vi "Walk Map.vi"(8 "error in (no error)":errorcluster, 11 "Map in":refnum<class "Maze.lvclass">) -> (3 "Map out":refnum<class "Maze.lvclass">)   [LabVIEW 2020, in "Maze.lvclass"]
uses:
  Maze.lvclass
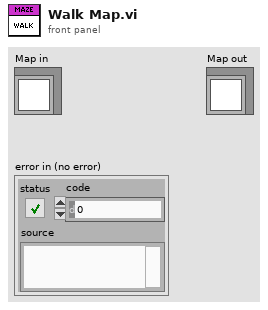
[diagram p1: front panel]
types:
  T1 = typedef "Maze.lvclass/Position.ctl" = cluster{"Row":u64, "Col":u64, "Next Move":enum16{"North", "East", "South", "West", "Halt"}}
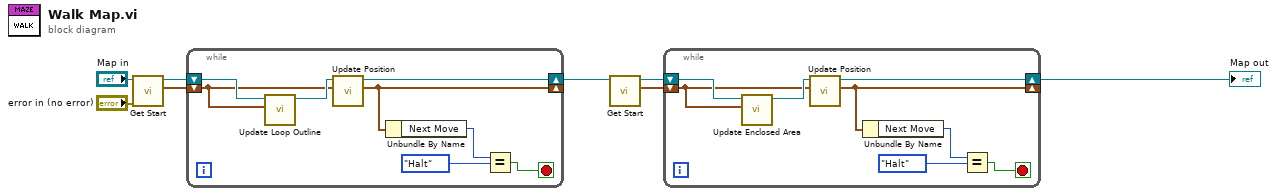
[diagram p0: block diagram]
diagram:
  n1 = call "Get Start.vi"("error in (no error)"="error in (no error)", "Map in"="Map in") -> ("Start Vectors"=w8:T1, "Map out"=w7:refnum<class "Maze.lvclass">)  [unwired: 7 in, 1 out]
  n2 = while {
    shift-right: [w15] -> _
    shift-left: w8 -> [w9]
    shift-right: [w12] -> w1
    shift-left: w7 -> [w11]
    stop <- w13 stop-if-true
    n3 = call "Update Loop Outline.vi"("Start Vectors"=w9, "Map in"=w11) -> ("Map out"=w10:refnum<class "Maze.lvclass">)  [unwired: 9 in]
    n4 = call "Update Position.vi"("Current"=w9, "Map In"=w10) -> ("Next"=w15:T1, "Map Out"=w12:refnum<class "Maze.lvclass">)  [unwired: 6 in, 2 out]
    n5 = Unbundle By Name(w15) -> ("Next Move"=w14:enum16{"North", "East", "South", "West", "Halt"})
    n6 = Equal?(x=w14, y=enum16{"North", "East", "South", "West", "Halt"}."Halt") -> (x = y?=w13:bool)
  }
  n7 = call "Get Start.vi"("Map in"=w1) -> ("Start Vectors"=w3:T1, "Map out"=w4:refnum<class "Maze.lvclass">)  [unwired: 8 in, 1 out]
  n8 = while {
    shift-right: [w23] -> _
    shift-left: w3 -> [w18]
    shift-right: [w17] -> w2
    shift-left: w4 -> [w20]
    stop <- w21 stop-if-true
    n9 = call "Update Enclosed Area.vi"("Start Vectors"=w18, "Map in"=w20) -> ("Map out"=w19:refnum<class "Maze.lvclass">)  [unwired: 9 in]
    n10 = call "Update Position.vi"("Current"=w18, "Map In"=w19) -> ("Next"=w23:T1, "Map Out"=w17:refnum<class "Maze.lvclass">)  [unwired: 6 in, 2 out]
    n11 = Unbundle By Name(w23) -> ("Next Move"=w22:enum16{"North", "East", "South", "West", "Halt"})
    n12 = Equal?(x=w22, y=enum16{"North", "East", "South", "West", "Halt"}."Halt") -> (x = y?=w21:bool)
  }
  "Map out" <- w2
